vi "SubVI_Find Circle #2.vi"(7 "功能":enum16{"半徑", "毛邊"}(ring), 8 "error in":errorcluster, 10 "Parameter_Circle":T2={"ROI Descriptor"={"Global Rectangle"=[], "Contours"=[]}, "Edge Options"={"Edge Options"={"Edge Polarity"=0, "Kernel Size"=3, "Width"=3, "Minimum Edge Strength"=10.0, "Interpolation Type"=enum."Bilinear Fixed", "Data Processing Method"=enum."Average"}, "Step Size"=3.0, "Scan Direction"=0, "Auto"=FALSE, "SD"=0.0}, "條件"={"半徑最大值"=0.0, "半徑最小值"=5.0}} {"Edge Options"."Scan Direction" items=["Outside To Inside", "Inside To Outside"]; "Edge Options"."Edge Options"."Edge Polarity" items=["All Edges", "Rising Edges", "Falling Edges"]; "Edge Options"."Edge Options"."Minimum Edge Strength" format="%.2f"; "Edge Options"."Edge Options"."Width" step=2; "Edge Options"."Edge Options"."Kernel Size" step=2; "ROI Descriptor"."Contours"."Type" items=["No Selection", "Point", "Line", "Rectangle", "Oval", "Polygon", "Free", "Annulus", "Unused2", "Unused3", "Broken Line", "Free Hand Line", "Rotated Rectangle"]}, 11 "Image in":T6) -> (0 "error out":errorcluster, 1 "Max & min":T1 {"Min Position"."Y" format="%.2f"; "Min Position"."X" format="%.2f"; "Max Position"."Y" format="%.2f"; "Max Position"."X" format="%.2f"}, 2 "Result_Circle":T5 {"Center"."Y" format="%.2f"; "Center"."X" format="%.2f"}, 3 "Image Out":T6)   [LabVIEW 2013]
uses:
  <vilib>/vision/Image Controls.llb/IMAQ Image.ctl
  Control/Control Find Circle #2.ctl
  <vilib>/vision/Measure.llb/Edge Options.ctl
  <vilib>/vision/Measure.llb/Edge Polarity.ctl
  <vilib>/Analysis/NI_AALBase.lvlib
  <vilib>/vision/NI_Vision_Development_Module.lvlib
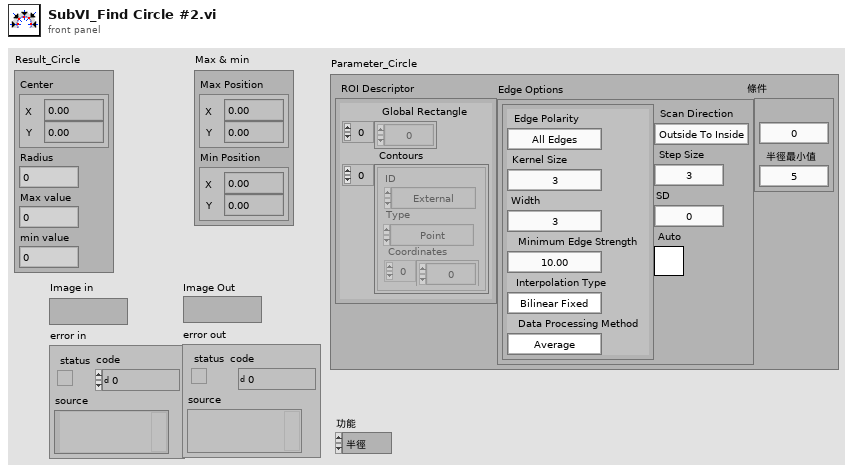
[diagram p1: front panel]
types:
  T1 = cluster{"Max Position":cluster{"X":sgl, "Y":sgl}, "Min Position":cluster{"X":sgl, "Y":sgl}}
  T2 = typedef "Control Find Circle #2.ctl" = cluster{"ROI Descriptor":cluster{"Global Rectangle":i32[], "Contours":cluster{"ID":enum32{"External", "Internal"}, "Type":u32, "Coordinates":i32[]}[]}, "Edge Options":cluster{"Edge Options":T3, "Step Size":dbl, "Scan Direction":u16, "Auto":bool, "SD":dbl}, "條件":cluster{"半徑最大值":dbl, "半徑最小值":dbl}}
  T3 = typedef "Edge Options.ctl" = cluster{"Edge Polarity":T4, "Kernel Size":u32, "Width":u32, "Minimum Edge Strength":sgl, "Interpolation Type":enum32{"Zero Order", "Bilinear", "Quadratic", "Cubic", "Bilinear Fixed"}, "Data Processing Method":enum32{"Average", "Median"}}
  T4 = typedef "Edge Polarity.ctl" = u32
  T5 = cluster{"Center":cluster{"X":sgl, "Y":sgl}, "Radius":dbl, "Max value":sgl, "min value":sgl}
  T6 = typedef "IMAQ Image.ctl" = refnum<image>
  T7 = cluster{"Center":cluster{"X":sgl, "Y":sgl}, "Radius":dbl}
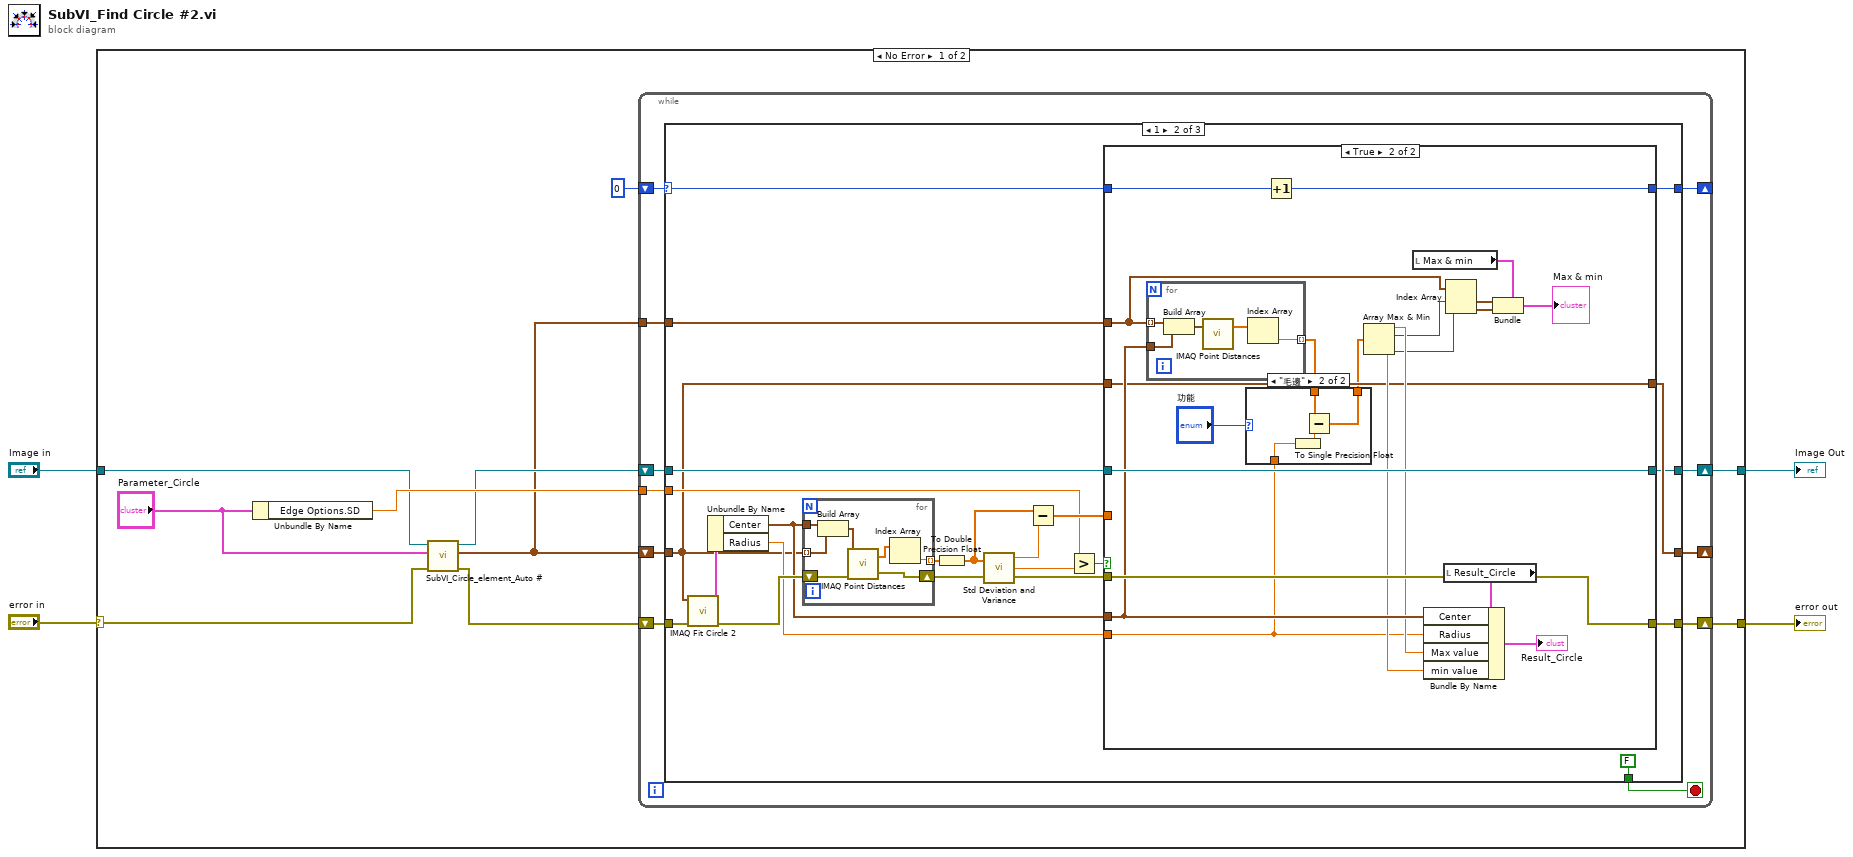
[diagram p0: block diagram]
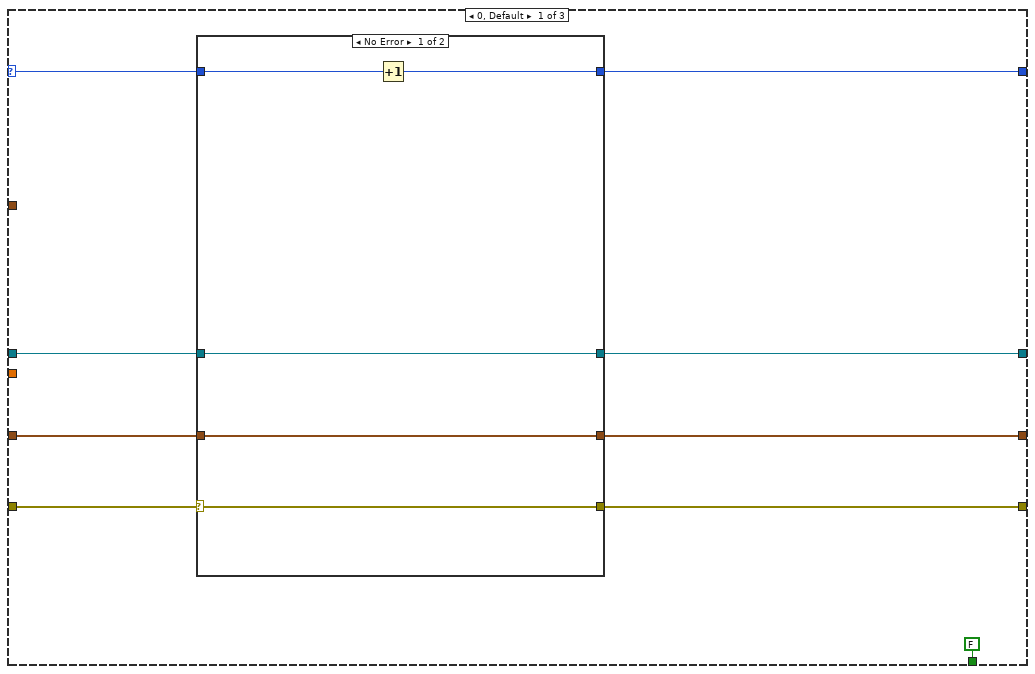
[diagram p2: hidden frame]
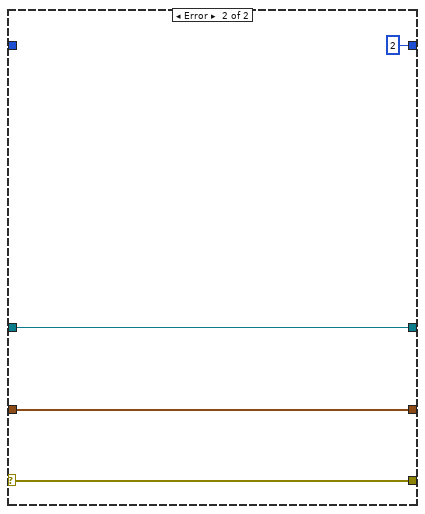
[diagram p3: hidden frame]
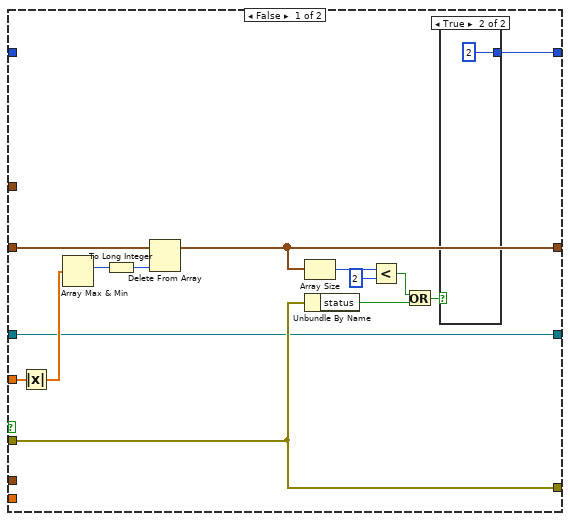
[diagram p4: hidden frame]
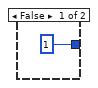
[diagram p5: hidden frame]
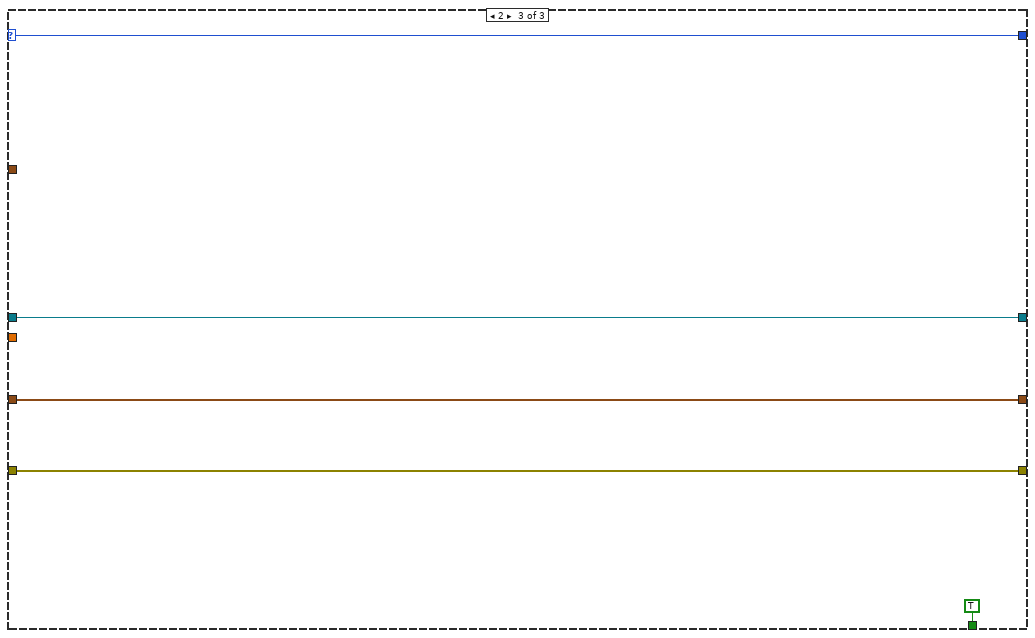
[diagram p7: hidden frame]
diagram:
  n1 = case shown="No Error" "error in" {
    selector: "error in" -> [w7 w126]
    tunnel: [w13 w126] -> w4
    tunnel: [w12 w125] -> w3
    tunnel: "Image in" -> [w9 w125]
    frame No Error {
      n2 = Unbundle By Name("Parameter_Circle") -> ("Edge Options.SD"=w11:dbl)
      n3 = call "SubVI_Circle_element_Auto #.vi"("Error In"=w7, "Parameter_Circle"="Parameter_Circle", "Image In"=w9) -> ("Error Out"=w8:errorcluster, "Location"=w5:cluster{"X":sgl, "Y":sgl}[], "Image Out"=w10:T6)  [unwired: 6 in]
      n4 = while {
        shift-right: [w23] -> _
        shift-left: 0 -> [w25]
        shift-right: [w22] -> w13
        shift-left: w8 -> [w24]
        shift-right: [w20] -> _
        shift-left: w5 -> [w21]
        shift-right: [w18] -> w12
        shift-left: w10 -> [w19]
        tunnel: w11 -> [w16]
        tunnel: w5 -> [w15]
        stop <- w17 stop-if-true
        n5 = case shown="1" w25 {
          selector: w25 -> [w30 w55 w121]
          tunnel: w24 -> [w28 w64 w120]
          tunnel: [w29 w56 w121] -> w23
          tunnel: [w32 w57 w120] -> w22
          tunnel: [w26 w61 w123] -> w20
          tunnel: w21 -> [w27 w45 w123]
          tunnel: w19 -> [w34 w60 w124]
          tunnel: [w33 w59 w124] -> w18
          tunnel: [FALSE FALSE TRUE] -> w17
          tunnel: w16 -> [_ w46 _]
          tunnel: w15 -> [_ w44 _]
          frame 0, Default {
            n6 = case shown="No Error" w28 {
              selector: w28 -> [w35 w41]
              tunnel: w34 -> [w36 w42]
              tunnel: [w36 w42] -> w33
              tunnel: [w35 w41] -> w32
              tunnel: w30 -> [w39 _]
              tunnel: [w38 2] -> w29
              tunnel: w27 -> [w37 w40]
              tunnel: [w37 w40] -> w26
              frame No Error {
                n7 = Increment(x=w39) -> (x+1=w38:i32)
              }
              frame Error {
              }
            }
          }
          frame 1 {
            n8 = call "IMAQ Fit Circle 2"("error in (no error)"=w64, "Radial Points"=w45) -> ("error out"=w63:errorcluster, "Circle"=w52:T7)  [unwired: 4 in, 4 out]
            n9 = Unbundle By Name(w52) -> ("Center"=w48:cluster{"X":sgl, "Y":sgl}, "Radius"=w47:dbl)
            n10 = for {
              tunnel: [w113] -> w51 mode=indexing
              shift-right: [w118] -> w58
              shift-left: w63 -> [w119]
              tunnel: w48 -> [w117]
              tunnel: w45 -> [w116] mode=indexing
              n11 = Build Array(w117, w116) -> (w115:cluster{"X":sgl, "Y":sgl}[])
              n12 = call "IMAQ Point Distances"("Points"=w115, "error in (no error)"=w119) -> ("Distances"=w114:sgl[], "error out"=w118:errorcluster)  [unwired: 3 in]
              n13 = Index Array(array=w114) -> (element=w113:sgl)  [unwired: 1 in]
            }
            n14 = To Double Precision Float(number=w51) -> (double precision float=w50:dbl[])
            n15 = call <vilib>:"Std Deviation and Variance.vi"("X"=w50) -> ("mean"=w49:dbl, "standard deviation"=w65:dbl)  [unwired: 1 in, 1 out]
            n16 = Subtract(x=w50, y=w49) -> (x-y=w54:dbl[])
            n17 = Greater?(x=w46, y=w65) -> (0:w62:bool)
            n18 = case shown="True" w62 {
              tunnel: w45 -> [w79 w91]
              tunnel: [w74 w91] -> w61
              tunnel: w60 -> [w66 w98]
              tunnel: [w66 w98] -> w59
              tunnel: w58 -> [w67 w97]
              tunnel: [w67 w97] -> w57
              tunnel: [w76 w101] -> w56
              tunnel: w55 -> [_ w102]
              tunnel: w54 -> [w68 _]
              tunnel: w48 -> [_ w96]
              tunnel: w47 -> [_ w84]
              tunnel: w44 -> [_ w86]
              frame False {
                n19 = Absolute Value(x=w68) -> (abs(x)=w69:dbl[])
                n20 = Array Max & Min(array=w69) -> (max index (indices)=w78:i32)  [unwired: 3 out]
                n21 = To Long Integer(number=w78) -> (32bit integer=w77:i32)
                n22 = Delete From Array(array=w79, index=w77) -> (array with subset deleted=w74:cluster{"X":sgl, "Y":sgl}[])  [unwired: 1 in, 1 out]
                n23 = Array Size(array=w74) -> (size(s)=w73:i32)
                n24 = Unbundle By Name(w67) -> ("status"=w75:bool)
                n25 = Less?(x=w73, y=2) -> (x < y?=w71:bool)
                n26 = Or(x=w71, y=w75) -> (x .or. y?=w70:bool)
                n27 = case shown="True" w70 {
                  tunnel: [1 2] -> w76
                  frame False {
                  }
                  frame True {
                  }
                }
              }
              frame True {
                n28 = for {
                  tunnel: w86 -> [w112] mode=indexing
                  tunnel: w96 -> [w111]
                  tunnel: [w108] -> w85 mode=indexing
                  n29 = Build Array(w112, w111) -> (w110:cluster{"X":sgl, "Y":sgl}[])
                  n30 = call "IMAQ Point Distances"("Points"=w110) -> ("Distances"=w109:sgl[])  [unwired: 4 in, 1 out]
                  n31 = Index Array(array=w109) -> (element=w108:sgl)  [unwired: 1 in]
                }
                n32 = case shown="\"毛邊\"" "功能" {
                  tunnel: w85 -> [w103 w107]
                  tunnel: w84 -> [_ w106]
                  tunnel: [w103 w105] -> w83
                  frame "半徑", Default {
                  }
                  frame "毛邊" {
                    n33 = To Single Precision Float(number=w106) -> (single precision float=w104:sgl)
                    n34 = Subtract(x=w107, y=w104) -> (x-y=w105:sgl[])
                  }
                }
                n35 = Increment(x=w102) -> (x+1=w101:i32)
                n36 = Array Max & Min(array=w83) -> (max value=w95:sgl, max index (indices)=w93:i32, min value=w94:sgl, min index (indices)=w92:i32)
                n37 = local read "Max & min"() -> (w87:T1)
                n38 = local read "Result_Circle"() -> (w100:T5)
                n39 = Bundle By Name(cluster=w100, "Center"=w96, "Radius"=w84, "Max value"=w95, "min value"=w94) -> (→"Result_Circle":T5)
                n40 = Index Array(array=w86, index #1=w93, index #2=w92) -> (element #1=w90:cluster{"X":sgl, "Y":sgl}, element #2=w89:cluster{"X":sgl, "Y":sgl})
                n41 = Bundle(cluster=w87, "Max Position"=w90, "Min Position"=w89) -> (→"Max & min":T1)
              }
            }
          }
          frame 2 {
          }
        }
      }
    }
    frame Error {
    }
  }
  "error out" <- w4
  "Image Out" <- w3
